vi "test10-StateChange_Event.vi"(8 "error in (no error)":errorcluster, 11 "TestCase in":refnum<class "testcase-CSMGlobalLog.lvclass">) -> (0 "error out":errorcluster, 3 "TestCase out":refnum<class "testcase-CSMGlobalLog.lvclass">)   [LabVIEW 2017, in "testcase-CSMGlobalLog.lvclass"]
uses:
  testcase-CSMGlobalLog.lvclass
  testcase-CSMGlobalLog.lvclass/testcase-CSMGlobalLog.ctl
  src/user.lib/_NEVSTOP/Communicable State Machine(CSM)/_Support/Typedef/_CSM_GlobalLog_MSG.ctl
  src/user.lib/_NEVSTOP/Communicable State Machine(CSM)/_Support/Typedef/_CSM_Response Source Message.ctl
  src/user.lib/_NEVSTOP/Communicable State Machine(CSM)/_Support/Typedef/_CSM_GlobalLog_MSG_TYPE.ctl
  24a778c7-405f-47d7-a6be-afdb60495ae4.vi
  src/user.lib/_NEVSTOP/Communicable State Machine(CSM)/_Support/GlobalEvent/GEvt-Generate with Rule Check.vi
  src/user.lib/_NEVSTOP/Communicable State Machine(CSM)/AdvanceAPI/CSM - Convert Error to Argument.vi
  src/user.lib/_NEVSTOP/Communicable State Machine(CSM)/_Support/GlobalEvent/Cache-GEvt Refs.vi
  src/user.lib/_NEVSTOP/Communicable State Machine(CSM)/AdvanceAPI/CSM - Make String Arguments Safe.vi
  src/user.lib/_NEVSTOP/Communicable State Machine(CSM)/_Support/ChangeFlag/FlagInstance-GEvt Refs.vi
  src/user.lib/_NEVSTOP/Communicable State Machine(CSM)/AdvanceAPI/CSM - Keywords.vi
  src/user.lib/_NEVSTOP/Communicable State Machine(CSM)/_Support/ChangeFlag/ChangeFlag-Read.vi
  src/user.lib/_NEVSTOP/Communicable State Machine(CSM)/_Support/ChangeFlag/ChangeFlagDB.vi
  src/user.lib/_NEVSTOP/Communicable State Machine(CSM)/_Support/GlobalEvent/FGV-GlobalEventRef(lvlibp).vi
  src/user.lib/_NEVSTOP/Communicable State Machine(CSM)/_Support/GlobalEvent/FGV-GlobalEventQueues(lvlibp).vi
  src/user.lib/_NEVSTOP/Communicable State Machine(CSM)/_Support/GlobalEvent/GEvt-Valid Subscribers.vi
  src/user.lib/_NEVSTOP/Communicable State Machine(CSM)/_Support/GlobalEvent/LogFilter/LogFilter - Check.vi
  src/user.lib/_NEVSTOP/Communicable State Machine(CSM)/_Support/GlobalEvent/LogFilter/LogFilter.lvclass
  <vilib>/addons/_JKI Toolkits/VI Tester/TestCase.llb/TestCase.lvclass
  src/user.lib/_NEVSTOP/Communicable State Machine(CSM)/Communicable State Machine.lvlib
  C:/Program Files (x86)/National Instruments/LabVIEW 2017/vi.lib/addons/_JKI Toolkits/VI Tester/TestCase.llb/TestCase.lvclass
panel:
  out "String Cache Each Loop":string
  out "LoopCount":i32
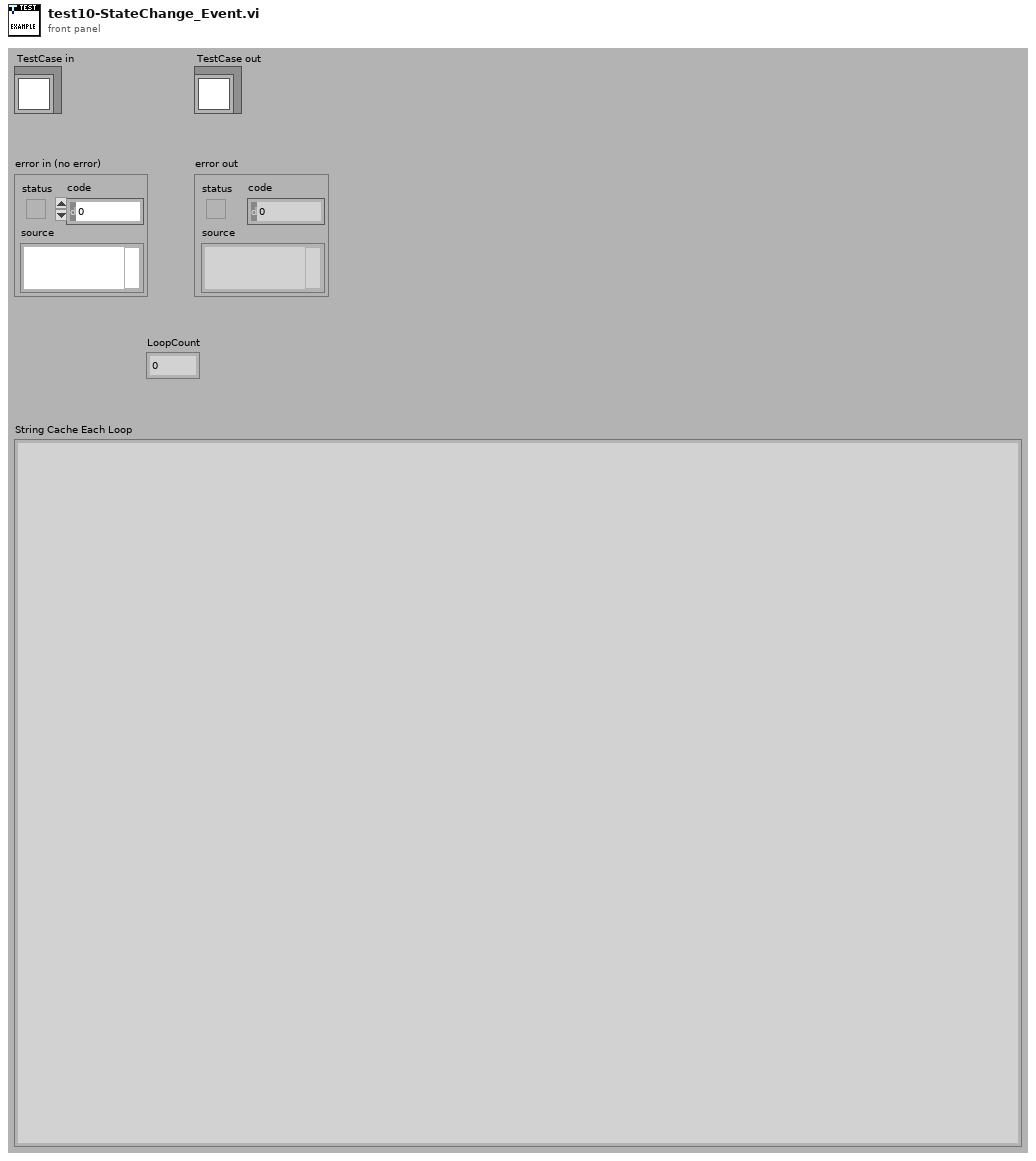
[diagram p1: front panel]
types:
  T1 = typedef "Communicable State Machine.lvlib/_CSM_GlobalLog_MSG.ctl" = cluster{"Name (\"\" to Use UUID)":string, "Current State":string, "Arguments":string, "Source Message":T2, "Source Module":string, "Complete(T)/Start(F)":bool, "LogType":T3, "Time Stamp":timestamp}
  T2 = typedef "Communicable State Machine.lvlib/_CSM_Response Source Message.ctl" = cluster{"‘State":string, "’Arguments":string, "’Error":errorcluster}
  T3 = typedef "Communicable State Machine.lvlib/_CSM_GlobalLog_MSG_TYPE.ctl" = enum16{"User Log", "State Change", "Status", "Interrupt", "Register", "Unregister", "Error Log", "Module Created", "Module Destroyed", "Async Message", "No-Rep Async Message", "Sync Message"}
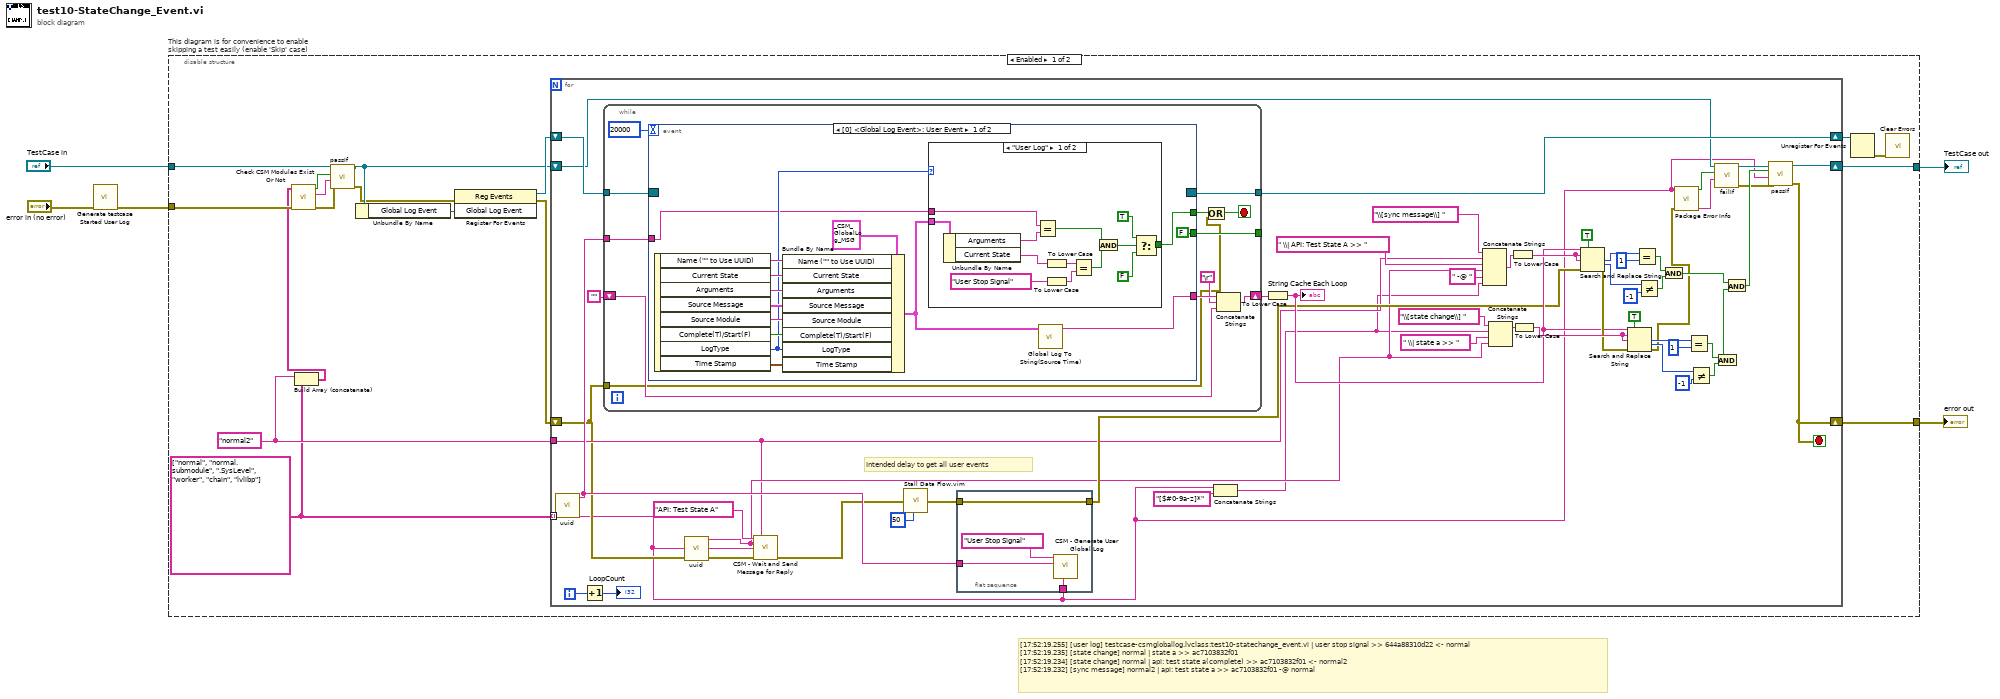
[diagram p0: block diagram]
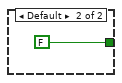
[diagram p2: hidden frame]
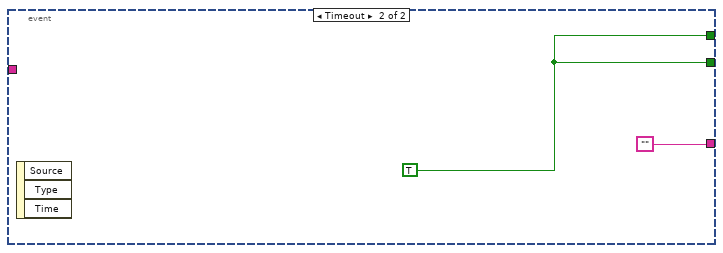
[diagram p3: hidden frame]
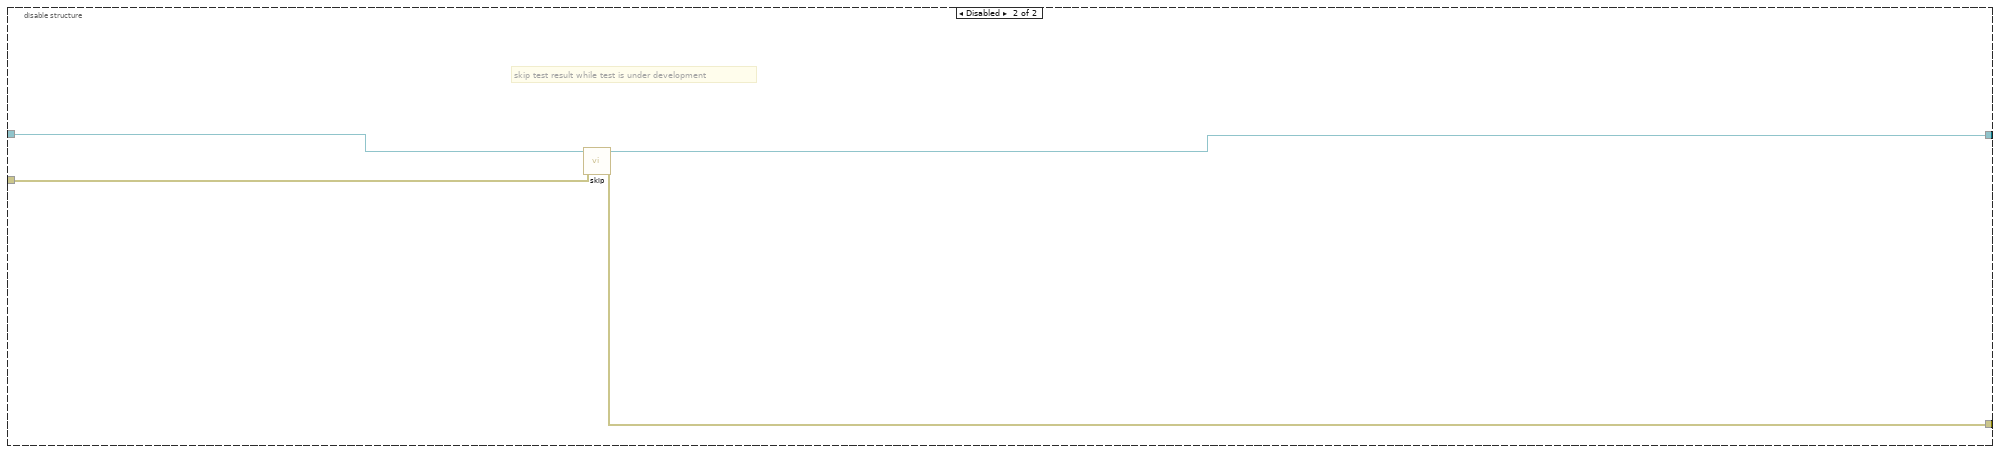
[diagram p4: hidden frame]
diagram:
  # "[17:52:19.255] [user log] testcase-csmgloballog.lvclass:test10-statechange_event.vi | user stop signal >> 644a88310d22 <- normal\n[17:52:19.235] [state change] normal | state a >> ac7103832f01\n[17:52:19.234] [state change] normal | api: test state a(complete) >> ac7103832f01 <- normal2\n[17:52:19.232] [sync message] normal2 | api: test state a >> ac7103832f01 -@ normal"
  n1 = call "Generate testcase Started User Log.vi"("Error In"="error in (no error)") -> ("error out"=w1:errorcluster)  [unwired: 10 in]
  n2 = disable-structure "This diagram is for convenience to enable skipping a test easily (enable 'Skip' case)" shown="Enabled" {
    disable-tunnel: "TestCase in" -> [w14 w126]
    disable-tunnel: [w18 w124] -> w2
    disable-tunnel: [w17 w125] -> w4
    disable-tunnel: w1 -> [w12 w123]
    frame Enabled {
      w11 = "normal2" ("CSM")
      w10 = string[] ["normal", "normal.submodule", ".SysLevel", "worker", "chain", "lvlibp"]
      n3 = Build Array (concatenate)(w11, w10) -> (w9:string[])
      n4 = call "Check CSM Modules Exist Or Not.vi"("error in"=w12, "CSM names in"=w9) -> ("error out"=w8:errorcluster, "Debug string"=w15:string, "All Modules Exist?"=w16:bool)  [unwired: 7 in]
      n5 = call-dynamic "passIf.vi"("error in (no error)"=w8, "message (\"\")"=w15, "pass"=w16, "TestCase in"=w14) -> ("error out"=w7:errorcluster, "TestCase out"=w13:refnum<class "testcase-CSMGlobalLog.lvclass">)  [unwired: 6 in]
      n6 = Unbundle By Name(w13) -> ("Global Log Event"=w22:refnum<user-event>)
      n7 = register-events(error in=w7, w22) -> (reference out=w21:refnum<event-registration>, error out=w19:errorcluster)  [unwired: 1 in]
      n8 = for {
        shift-right: [w75] -> w20
        shift-left: w21 -> [w76]
        shift-right: [w71] -> w17
        shift-left: w19 -> [w30]
        tunnel: w10 -> [w23] mode=indexing
        shift-right: [w74] -> w18
        shift-left: w13 -> [w24]
        tunnel: w11 -> [w32]
        i -> [w73]
        stop <- w71 stop-if-true
        # "Intended delay to get all user events"
        n9 = call "uuid.vi"() -> ("UUID"=w70:string)  [unwired: 11 in]
        n10 = Increment(x=w73) -> (x+1=→"LoopCount":i32)
        n11 = while {
          tunnel: w76 -> [w92]
          tunnel: [w91] -> w75
          shift-right: [w85] -> w67
          shift-left: "" -> [w87]
          tunnel: w70 -> [w89]
          tunnel: [w88] -> _
          tunnel: w30 -> [w81]
          stop <- w83 stop-if-true
          n12 = event shown="[0] <Global Log Event>: User Event" {
            selector: w92 -> [_ _]
            dyn-events: [_ _] -> w91
            timeout: 20000 -> [_ _]
            tunnel: [w93 ""] -> w86
            tunnel: [w95 w122] -> w82
            tunnel: w89 -> [w96 _]
            tunnel: [FALSE ("Stop") w122] -> w88
            event User Event {
              n13 = event-data() -> ("Name (\"\" to Use UUID)"=w105:string, "Current State"=w104:string, "Arguments"=w103:string, "Source Message"=w102:T2, "Source Module"=w101:string, "Complete(T)/Start(F)"=w100:bool, "LogType"=w97:T3, "Time Stamp"=w99:timestamp)  [unwired: 1 in]
              n14 = Bundle By Name(cluster=T1 {"Name (\"\" to Use UUID)"="", "Current State"="", "Arguments"="", "Source Message"={"‘State"="", "’Arguments"="", "’Error"={"status"=FALSE, "code"=0, "source"=""}}, "Source Module"="", "Complete(T)/Start(F)"=FALSE, "LogType"=enum."State Change", "Time Stamp"=timestamp(0 s since 1904-01-01)} ("Cross CSM Data"), "Name (\"\" to Use UUID)"=w105, "Current State"=w104, "Arguments"=w103, "Source Message"=w102, "Source Module"=w101, "Complete(T)/Start(F)"=w100, "LogType"=w97, "Time Stamp"=w99) -> (w94:T1)
              n15 = case shown="\"User Log\"" w97 {
                tunnel: w94 -> [w119 _]
                tunnel: w96 -> [w118 _]
                tunnel: [w107 FALSE] -> w95
                frame "User Log" {
                  n16 = Unbundle By Name(w119) -> ("Arguments"=w117:string, "Current State"=w116:string)
                  n17 = Equal?(x=w118, y=w117) -> (x = y?=w111:bool)
                  n18 = To Lower Case(string=w116) -> (all lower case string=w115:string)
                  n19 = To Lower Case(string="User Stop Signal" ("Log")) -> (all lower case string=w113:string)
                  n20 = Equal?(x=w115, y=w113) -> (x = y?=w112:bool)
                  n21 = And(x=w111, y=w112) -> (x .and. y?=w110:bool)
                  n22 = Select(t=TRUE, s=w110, f=FALSE) -> (s? t:f=w107:bool)
                }
                frame Default {
                }
              }
              n23 = call "Global Log To String(Source Time).vi"("Log"=w94) -> ("Log String"=w93:string)  [unwired: 9 in]
            }
            event Timeout {
              w122 = TRUE ("Stop")
              n24 = event-data() -> ()  [unwired: 1 in, 3 out]
            }
          }
          n25 = Or(x=w82, y=w81) -> (x .or. y?=w83:bool)
          n26 = Concatenate Strings(w86, "\r", w87) -> (w85:string)
        }
        n27 = call "uuid.vi"() -> ("UUID"=w36:string)  [unwired: 11 in]
        n28 = call "CSM - Wait and Send Message for Reply.vi"("State"="API: Test State A", "Current Module (\"\" to Generate an ID)"=w32, "Arguments (\"\")"=w36, "Target Module"=w23, "Error In (No Error)"=w30) -> ("error out"=w65:errorcluster)  [unwired: 7 in, 3 out]
        n29 = call "Stall Data Flow.vim"("value in"=w65, "milliseconds to wait"=u32 50) -> ("value out"=w68:errorcluster)  [unwired: 1 out]
        n30 = flat-sequence {
          tunnel: w68 -> [w77]
          tunnel: [w77] -> w37
          tunnel: w70 -> [w79]
          tunnel: w23 -> [w78]
          frame #0 {
            n31 = call "CSM - Generate User Global Log.vi"("From Who"=w78, "Arguments"=w79, "Log"="User Stop Signal") -> ()  [unwired: 8 in, 1 out]
          }
        }
        n32 = Concatenate Strings(w23, "[$#0-9a-z]*" ("string")) -> (w31:string)
        n33 = To Lower Case(string=w67) -> (all lower case string=w39:string)
        "String Cache Each Loop" <- w39
        n34 = Concatenate Strings("\\[sync message\\] " ("regular expression"), w32, " \\| API: Test State A >> " ("string"), w36, " -@ " ("string"), w31) -> (w61:string)
        n35 = Concatenate Strings("\\[state change\\] " ("regular expression"), w31, " \\| state a >> " ("string"), w36) -> (w63:string)
        n36 = To Lower Case(string=w61) -> (all lower case string=w59:string)
        n37 = To Lower Case(string=w63) -> (all lower case string=w48:string)
        n38 = Search and Replace String(replace all?=TRUE ("replace all? (F)"), input string=w39, search string=w59, replace string=w59, error in=w37) -> (number of replacements=w58:i32, offset past replacement=w57:i32, error out=w47:errorcluster)  [unwired: 3 in, 1 out]
        n39 = Search and Replace String(replace all?=TRUE ("replace all? (F)"), input string=w39, search string=w48, replace string=w48, error in=w47) -> (number of replacements=w50:i32, offset past replacement=w51:i32, error out=w27:errorcluster)  [unwired: 3 in, 1 out]
        n40 = Equal?(x=w58, y=1) -> (x = y?=w55:bool)
        n41 = Not Equal?(x=w57, y=-1) -> (x != y?=w54:bool)
        n42 = And(x=w55, y=w54) -> (x .and. y?=w41:bool)
        n43 = call "Package Error Info.vi"("error in"=w27, "String in"=w23) -> ("packed error info out"=w28:string, "error status"=w29:bool)  [unwired: 8 in]
        n44 = Equal?(x=w50, y=1) -> (x = y?=w52:bool)
        n45 = Not Equal?(x=w51, y=-1) -> (x != y?=w53:bool)
        n46 = call-dynamic "failIf.vi"("message (\"\")"=w28, "fail"=w29, "TestCase in"=w24) -> ("error out"=w26:errorcluster, "TestCase out"=w25:refnum<class "testcase-CSMGlobalLog.lvclass">)  [unwired: 7 in]
        n47 = And(x=w52, y=w53) -> (x .and. y?=w46:bool)
        n48 = And(x=w41, y=w46) -> (x .and. y?=w34:bool)
        n49 = call-dynamic "passIf.vi"("error in (no error)"=w26, "message (\"\")"=w23, "pass"=w34, "TestCase in"=w25) -> ("error out"=w71:errorcluster, "TestCase out"=w74:refnum<class "testcase-CSMGlobalLog.lvclass">)  [unwired: 6 in]
      }
      n50 = Unregister For Events(event registration refnum=w20) -> (error out=w6:errorcluster)  [unwired: 1 in]
      n51 = call <vilib>:"Clear Errors.vi"("error in (no error)"=w6) -> ()  [unwired: 5 in, 2 out]
    }
    frame Disabled {
      # "skip test result while test is under development"
      n52 = call <vilib>:"skip.vi"("error in (no error)"=w123, "TestCase in"=w126) -> ("error out"=w125:errorcluster, "TestCase out"=w124:refnum<class "testcase-CSMGlobalLog.lvclass">)  [unwired: 8 in]
    }
  }
  "error out" <- w4
  "TestCase out" <- w2
